vi "Configure Start Trigger.vi"(0 "Register Bus":T2, 1 "scope":string(combo)="rx", 5 "start trigger":T1 caption="Start Trigger", 11 "error in":errorcluster) -> (4 "Register Bus (out)":T2, 15 "error out":errorcluster)   [LabVIEW 2017]
doc: "Configure the device's start trigger by selecting the trigger source.\n\n<B>Input Parameters</B>\n\n<B>Register Bus</B> The Register Bus object created by the ni579x Open VI and used as the session handle for the NI-579x Configuration Design Library.\n\n<B>scope</B> is the channel to configure a start trigger for. The options are \"rx\" and \"tx\".\n\n<B>start trigger</B> is the trigger to use to start the stream circuit on the device.\n\n<B>error in</B> describes error conditions that occur before this node runs. This input provides standard 'error in' functionality.\n\n<B>Output Parameters</B>\n\n<B>Register Bus (out)</B> The Register Bus object created by the ni579x Open VI and used as the session handle for the NI-579x Configuration Design Library.\n\n<B>error out</B> contains error information. This output provides standard 'error out' functionality."
uses:
  <instrlib>/_niInstr/Register Bus/v0/Host/Public/Register Bus Session.ctl
  <instrlib>/_niInstr/Register Bus/v0/Host/Private/Session Data.ctl
  Start Trigger.ctl
  Rx FPGA VI Reference.ctl
  Tx FPGA VI Reference.ctl
  <vilib>/Utility/error.llb/Error Cluster From Error Code.vi
  <vilib>/rvi/errors/niLvFpgaAdjustHostInterfaceError.vi
  <vilib>/ErrorRing/Error Ring.xnode
  <vilib>/rvi/interface/nirviReadWriteControl/nirviReadWriteControl.xnode
  NiFpgaLv.dll
  <vilib>/rvi/interface/Simulation/niFpgaSimulationCallBeginRW.vi
  <instrlib>/_niInstr/Register Bus/v0/Host/niInstr Register Bus v0 Host.lvlib
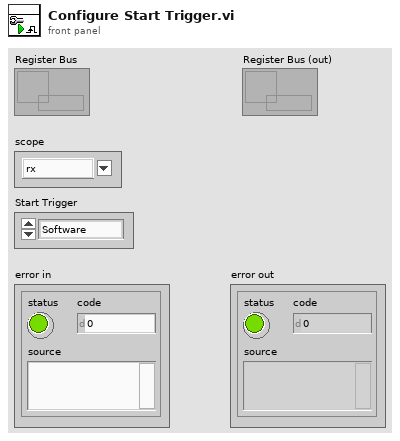
[diagram p1: front panel]
types:
  T1 = typedef "Start Trigger.ctl" = enum8{"Software", "Digital Edge", "Rx Start Trigger", "Tx Start Trigger"}
  T2 = typedef "niInstr Register Bus v0 Host.lvlib/Register Bus Session.ctl" = refnum<queue>
  T3 = typedef "Rx FPGA VI Reference.ctl" = refnum<k20>
  T4 = typedef "Tx FPGA VI Reference.ctl" = refnum<k20>
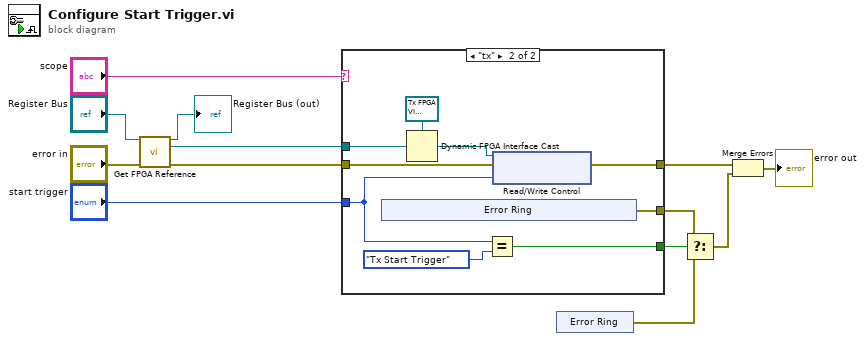
[diagram p0: block diagram]
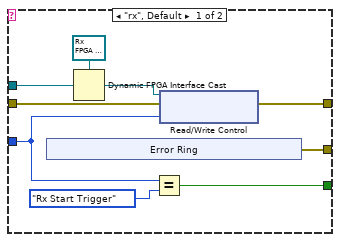
[diagram p2: hidden frame]
diagram:
  n1 = call <instrlib>:"Get FPGA Reference.vi"("session in"="Register Bus", "error in"="error in") -> ("session out"=→"Register Bus (out)":T2, "fpga ref"=w10:refnum<k20>, "error out"=w11:errorcluster)  [unwired: 11 in]
  n2 = case shown="\"tx\"" "scope" {
    tunnel: "start trigger" -> [w17 w31]
    tunnel: w10 -> [w22 w36]
    tunnel: [w19 w33] -> w3
    tunnel: w11 -> [w18 w32]
    tunnel: [w15 w29] -> w5
    tunnel: [w14 w28] -> w4
    frame "rx", Default {
      n3 = xnode ("Error Ring")() -> ("error out"=w14:errorcluster)
      n4 = Dynamic FPGA Interface Cast(Session In=T3 refnum ("FPGA VI Reference Out"), Type=w22) -> (Session Out=w20:T3)
      n5 = Equal?(x=w17, y=Start_Trigger."Rx Start Trigger" ("start trigger")) -> (x = y?=w15:bool)
      n6 = xnode "Read/Write Control"("FPGA VI Reference In"=w20, "error in"=w18, "rx.trigger select"=w17) -> ("error out"=w19:errorcluster)  [unwired: 1 out]
    }
    frame "tx" {
      n7 = xnode "Error Ring"() -> ("error out"=w28:errorcluster)
      n8 = Dynamic FPGA Interface Cast(Session In=T4 refnum ("FPGA VI Reference Out"), Type=w36) -> (Session Out=w34:T4)
      n9 = Equal?(x=w31, y=Start_Trigger."Tx Start Trigger" ("start trigger")) -> (x = y?=w29:bool)
      n10 = xnode "Read/Write Control"("FPGA VI Reference In"=w34, "error in"=w32, "tx.trigger select"=w31) -> ("error out"=w33:errorcluster)  [unwired: 1 out]
    }
  }
  n11 = xnode "Error Ring"() -> ("error out"=w6:errorcluster)
  n12 = Select(t=w4, s=w5, f=w6) -> (s? t:f=w1:errorcluster)
  n13 = Merge Errors(w3, w1) -> (→"error out":errorcluster)
